vi "clean_providers.vi"(8 "error in (no error)":errorcluster, 11 "system.logging in":refnum<class "system.logging.lvclass">) -> (0 "error out":errorcluster, 3 "system.logging out":refnum<class "system.logging.lvclass">)   [LabVIEW 2021, in "system.logging.lvclass"]
uses:
  system.logging.lvclass
  system.logging.lvclass/system.logging.ctl
  system.logging.provider/system.logging.provider.lvclass
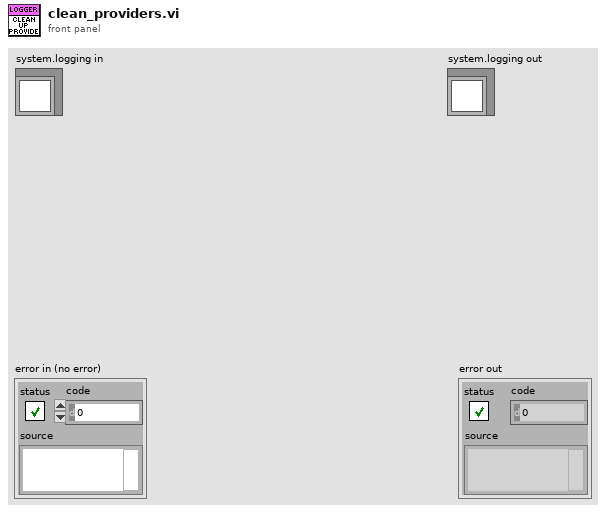
[diagram p1: front panel]
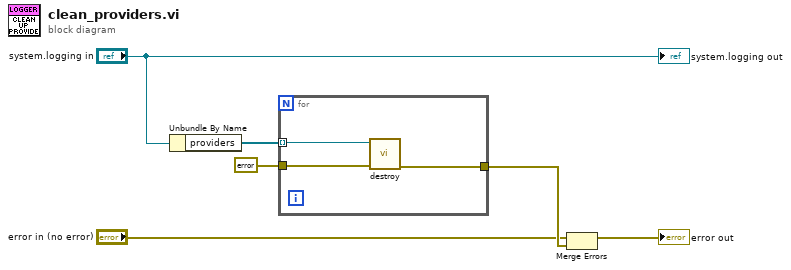
[diagram p0: block diagram]
diagram:
  n1 = Unbundle By Name("system.logging in") -> ("providers"=w5:refnum<class "system.logging.provider.lvclass">[])
  n2 = for {
    tunnel: w5 -> [w9] mode=indexing
    tunnel: [w8] -> w4
    tunnel: errorcluster {"status"=FALSE, "code"=0, "source"=""} ("error in (no error)") -> [w7]
    n3 = call-dynamic "destroy.vi"("error in (no error)"=w7, "system.logging.provider in"=w9) -> ("error out"=w8:errorcluster)  [unwired: 9 in]
  }
  n4 = Merge Errors("error in (no error)", w4) -> (→"error out":errorcluster)
  "system.logging out" <- "system.logging in"
